vi "TestExplicitMessgaes.vi"() -> ()   [LabVIEW 2022 SP3, in "TopLevel.lvclass"]
uses:
  TopLevel/TopLevel.lvclass
  Typedefs/SetExplicitMessage API Data.ctl
  Typedefs/Motor Controller Parameter-Set.ctl
  <vilib>/ethernetip/ethernetip.llb/ethernetip.ctl
  C:/projects/Digilens_IPLC/Classes/Motor Controller/EEIP.dll
  EEIP.dll
  Motor Controller.lvclass
  <vilib>/ethernetip/ethernetip.lvlib
panel:
  in  "SendCmd 2":bool
  in  "SetExplicitMessage API Data LV":T1={"Motor Controller Parameter"=enum."Home Stage", "value"=0}
  out "Return":cluster{"size":i32, "GetAttributeSingle":u8[]}
  in  "SendCmd":bool
  in  "SetExplicitMessage API Data":T1={"Motor Controller Parameter"=enum."Home Stage", "value"=0}
  in  "OK":bool
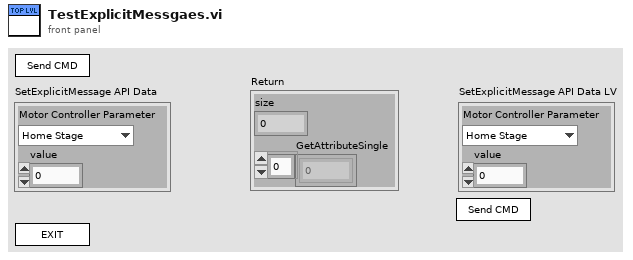
[diagram p1: front panel]
types:
  T1 = typedef "Motor Controller.lvclass/SetExplicitMessage API Data.ctl" = cluster{"Motor Controller Parameter":T2, "value":i32}
  T2 = typedef "Motor Controller.lvclass/Motor Controller Parameter-Set.ctl" = enum16{"Print Speed", "Jog Speed", "PR Path", "Enable Servo", "Disable Servo", "Move Stage to Under PH1", "Move Stage to Under PH2", "Move Stage to Under PH3", "Move Stage to Under PH4", "Move Stage to Under PH5", "Move Stage to Under PH6", "Home Stage", "Return Stage to 0", "Print Stage", "Write Speed", "Write Index", "Stop Stage"}
  T3 = enum32{"Invalid", "Standard", "Closed", "Hidden", "Minimized", "Maximized"}
  T4 = enum32{"invalid app kind", "Development System", "Run Time System", "Student Edition", "Embedded LabVIEW", "Evaluation", "Custom"}
  T5 = typedef "ethernetip.lvlib/ethernetip.ctl" = refnum<k21>
  T6 = cluster{"Core":cluster{"Current VI Reference":refnum<vi>, "Close Panel on Exit?":bool}, ".NET Refnum":refnum<k24>, "Session out":T5}
  T7 = cluster{"Current VI Reference":refnum<vi>, "Close Panel on Exit?":bool}
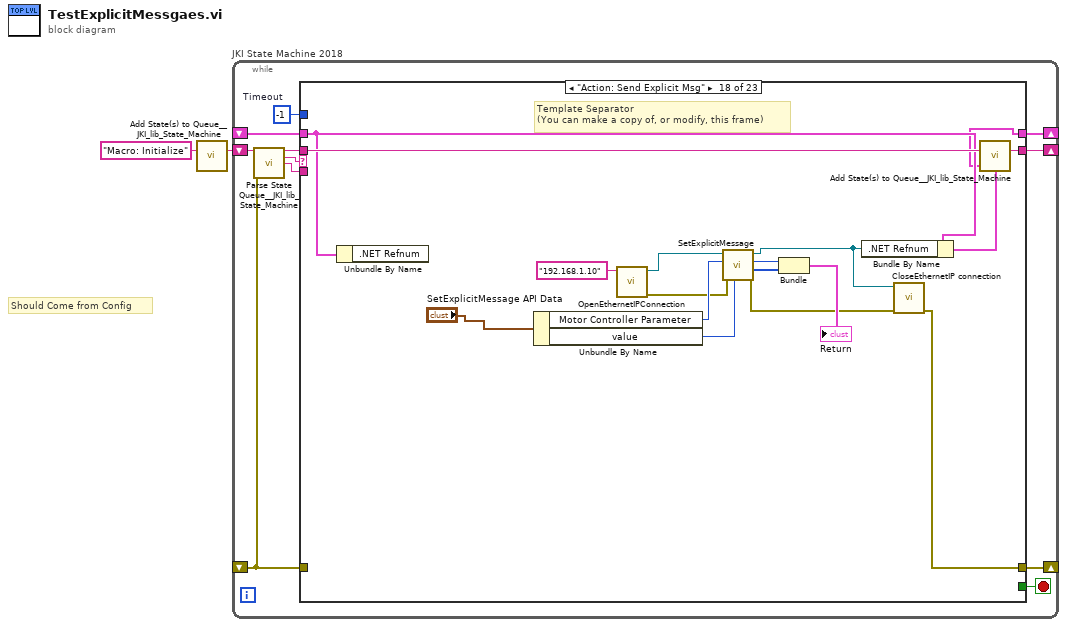
[diagram p0: block diagram]
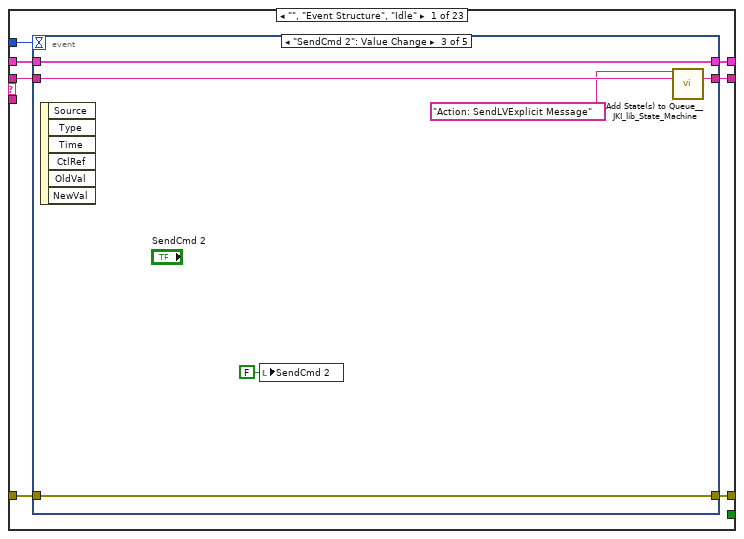
[diagram p2: hidden frame]
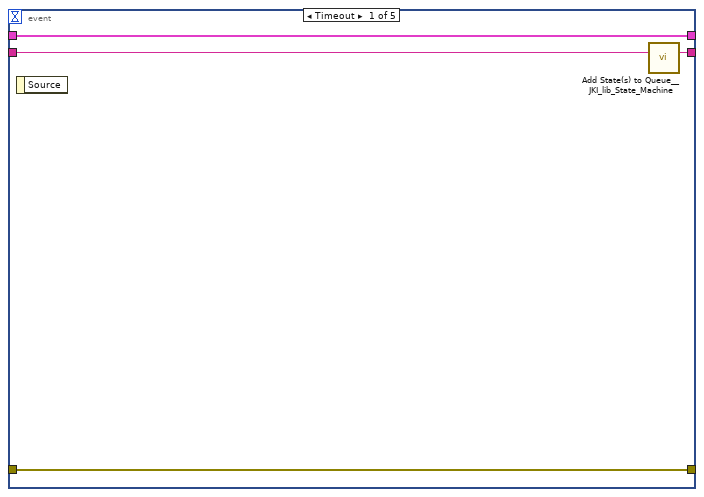
[diagram p3: hidden frame]
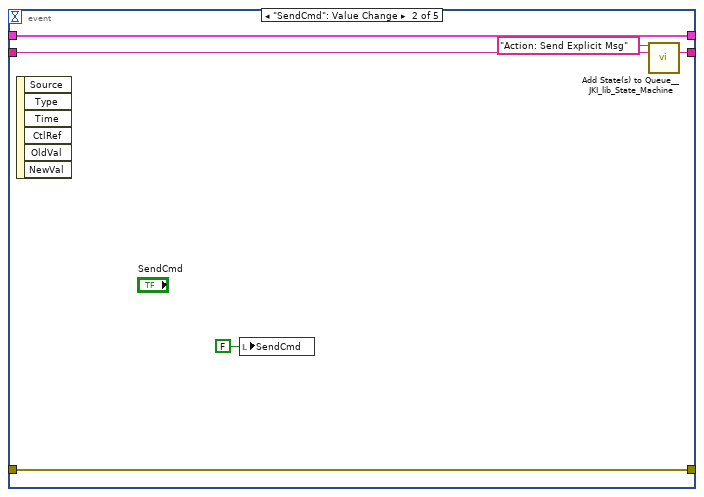
[diagram p4: hidden frame]
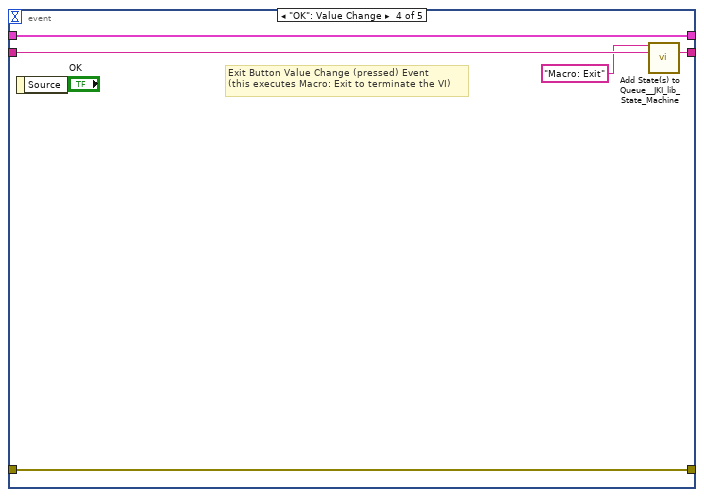
[diagram p5: hidden frame]
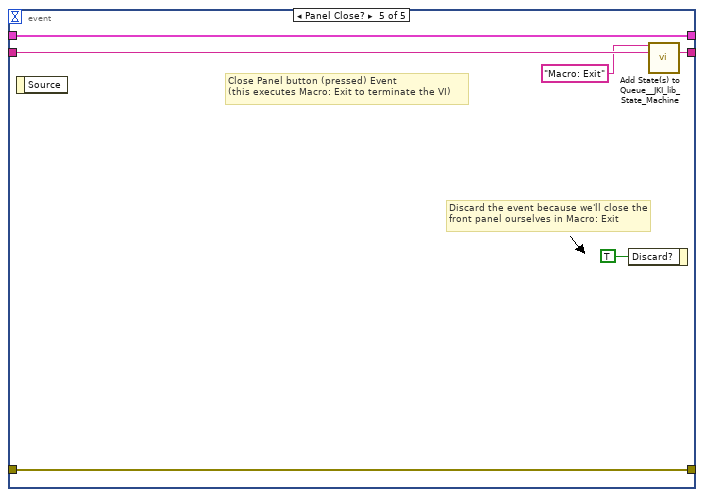
[diagram p6: hidden frame]
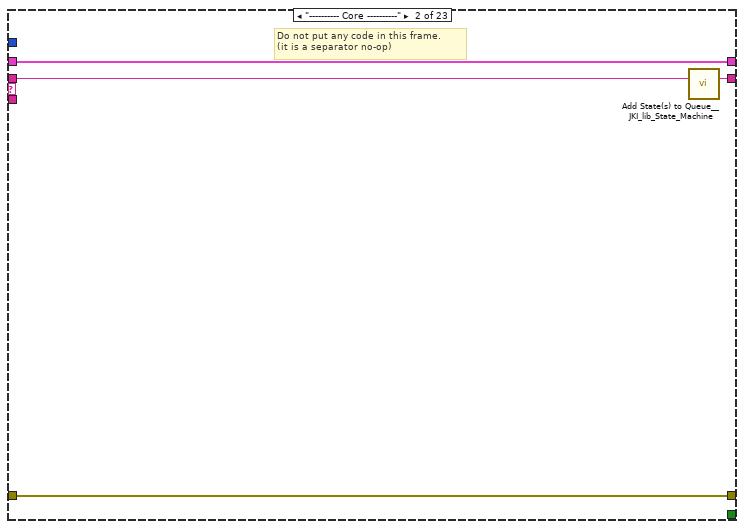
[diagram p7: hidden frame]
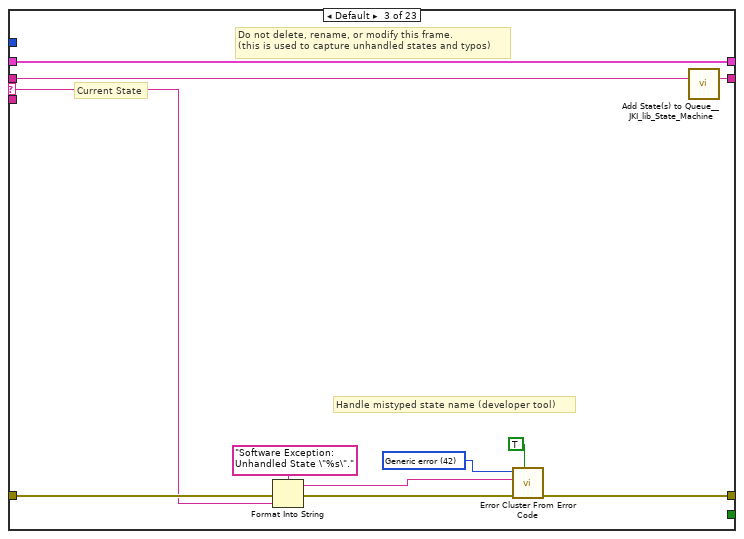
[diagram p8: hidden frame]
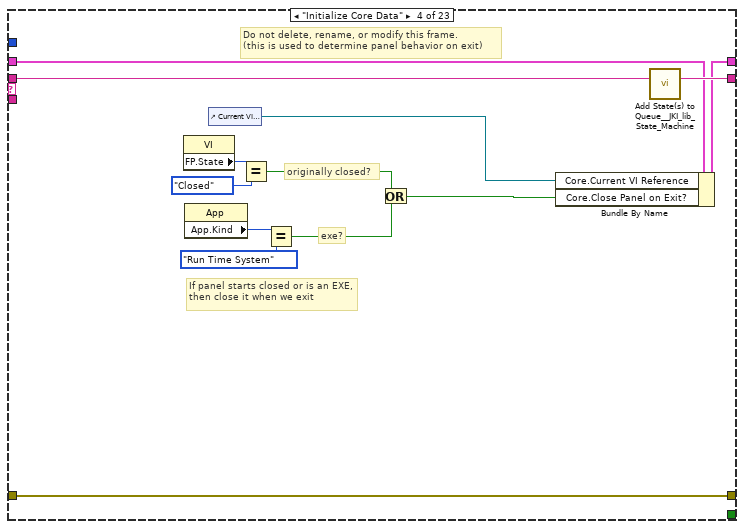
[diagram p9: hidden frame]
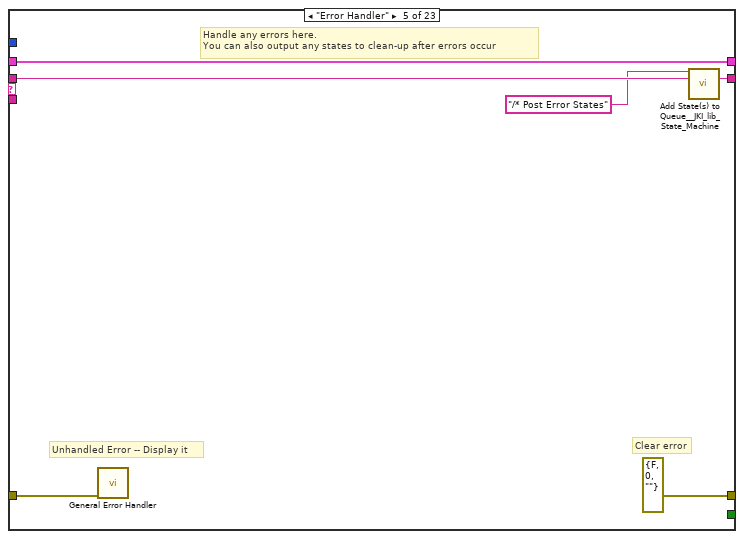
[diagram p10: hidden frame]
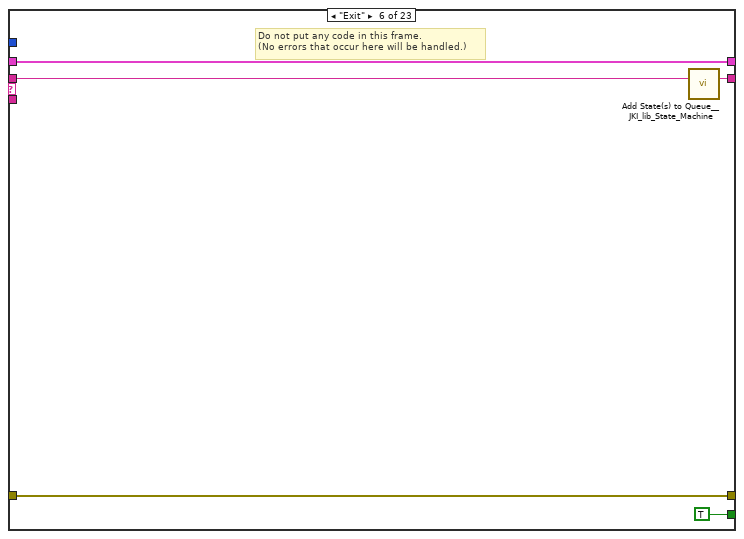
[diagram p11: hidden frame]
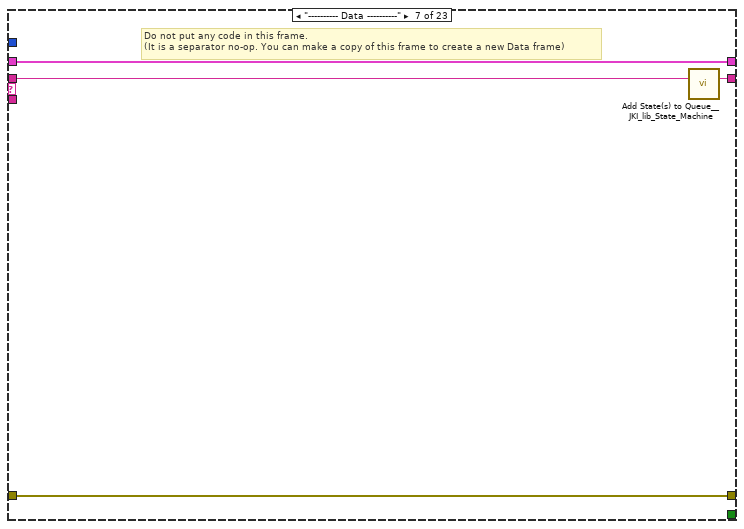
[diagram p12: hidden frame]
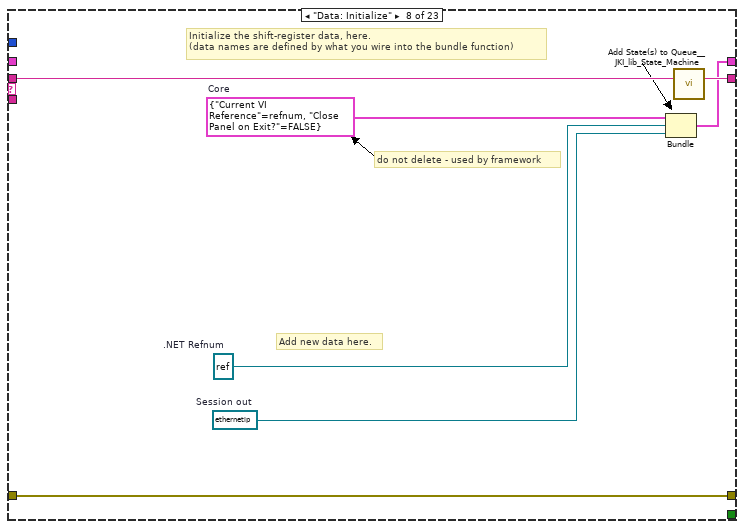
[diagram p13: hidden frame]
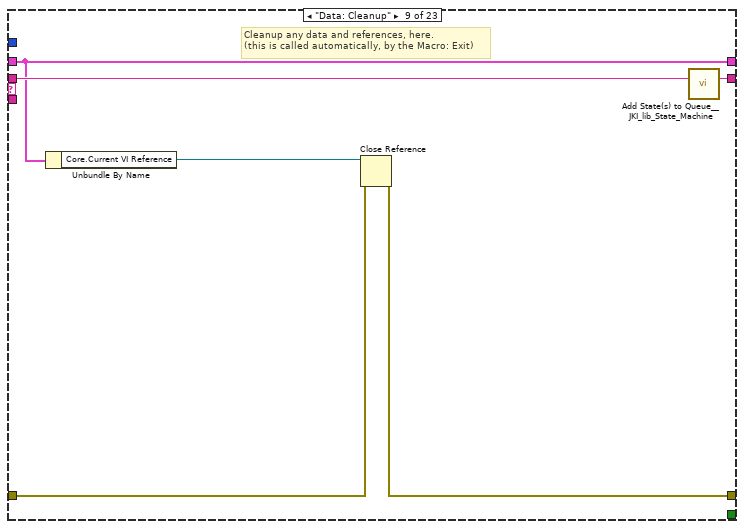
[diagram p14: hidden frame]
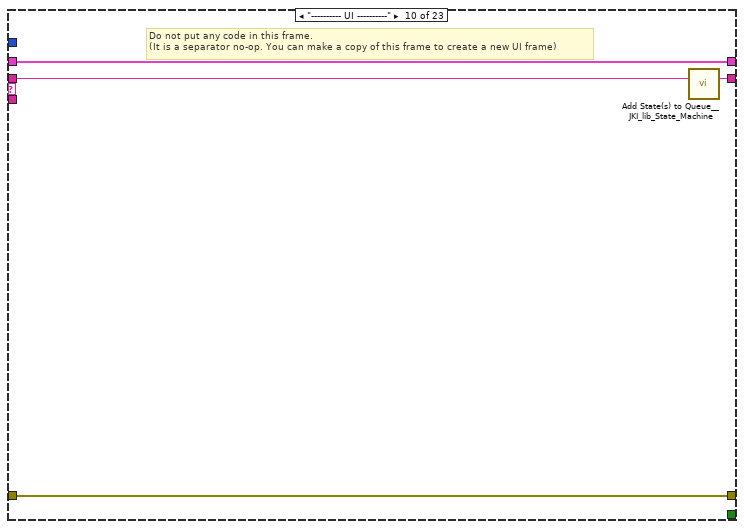
[diagram p15: hidden frame]
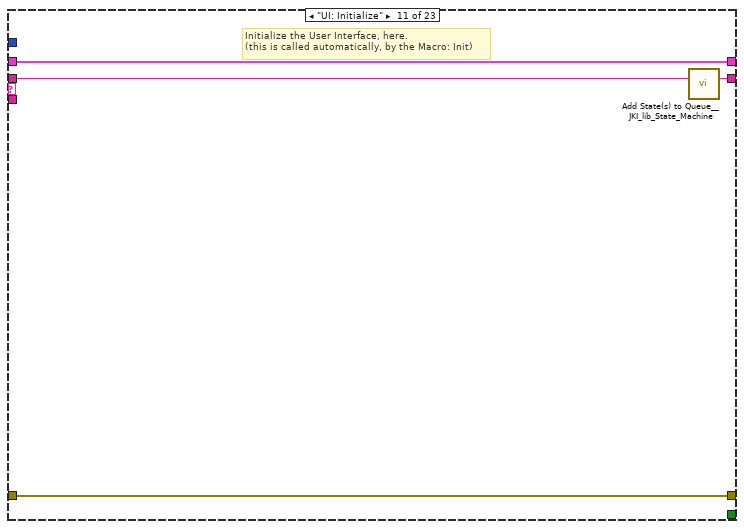
[diagram p16: hidden frame]
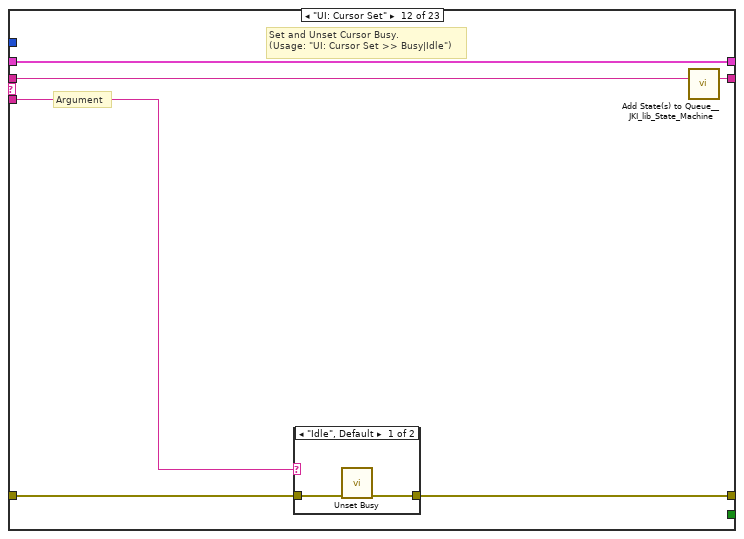
[diagram p17: hidden frame]
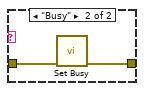
[diagram p18: hidden frame]
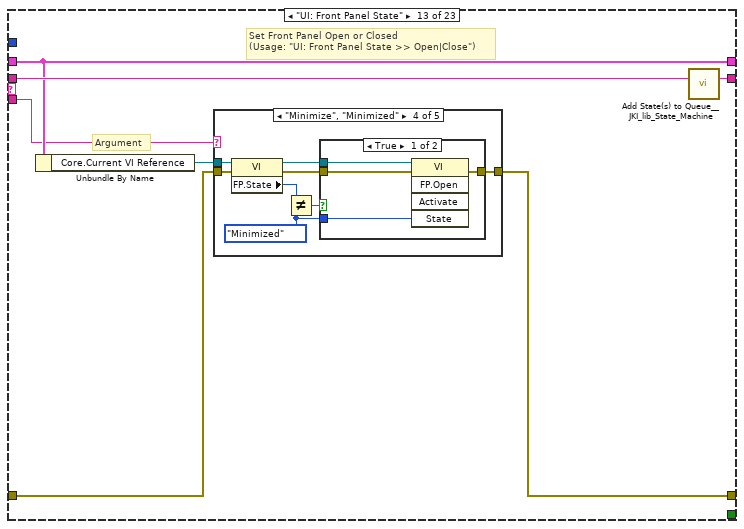
[diagram p19: hidden frame]
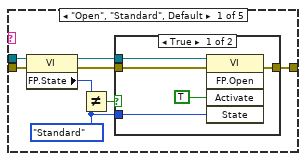
[diagram p20: hidden frame]
diagram:
  # "Should Come from Config"
  n1 = call <vilib>:"Add State(s) to Queue__JKI_lib_State_Machine.vi"("State(s) in (\"\")"="Macro: Initialize") -> ("States Out"=w2:string)  [unwired: 14 in]
  n2 = while "JKI State Machine 2018" {
    shift-right: [w6] -> _
    shift-left: _ -> [w5]
    shift-right: [w9] -> _
    shift-left: _ -> [w3]
    shift-right: [w8] -> _
    shift-left: w2 -> [w10]
    stop <- w7 stop-if-true
    w4 = -1  # Timeout
    n3 = call <vilib>:"Parse State Queue__JKI_lib_State_Machine.vi"("State Queue"=w10, "Error In (no error)"=w3) -> ("Remaining States"=w12:string, "Current State"=w13:string, "Arguments"=w11:string)  [unwired: 11 in]
    n4 = case shown="\"Action: Send Explicit Msg\"" w13 {
      selector: w13 -> [_ _ w52 _ _ _ _ _ _ _ _ _ _ _ _ _ _ _ _ _ _ _ _]
      tunnel: w12 -> [w20 w51 w56 w75 w81 w86 w90 w97 w103 w107 w111 w117 w128 w197 w202 w212 w216 w232 w243 w252 w261 w267 w273]
      tunnel: w11 -> [_ _ _ _ _ _ _ _ _ _ _ w112 w122 _ _ _ _ _ _ _ _ _ _]
      tunnel: w5 -> [w18 w48 w54 w68 w78 w84 w87 _ w98 w104 w109 w115 w124 w194 w199 w209 w213 w226 w241 w246 w258 w264 w271]
      tunnel: [w17 w49 w58 w72 errorcluster {"status"=FALSE, "code"=0, "source"=""} ("error out") w83 w88 w94 w99 w105 w108 w113 w125 w195 w200 w210 w214 w218 w236 w245 w257 w263 w268] -> w9
      tunnel: w3 -> [w16 w49 w57 w72 w77 w83 w88 w94 w100 w105 w108 w114 w126 w195 w200 w210 w214 _ w234 w244 w256 w262 w269]
      tunnel: [w19 w50 w55 w74 w80 w85 w89 w96 w102 w106 w110 w116 w127 w196 w201 w211 w215 w231 w242 w251 w260 w266 w272] -> w8
      tunnel: [_ _ _ _ _ TRUE _ _ _ _ _ _ _ _ _ _ _ _ _ _ _ _ _] -> w7
      tunnel: [w15 w48 w54 w73 w78 w84 w87 w95 w98 w104 w109 w115 w124 w194 w199 w209 w213 w225 w240 w247 w259 w264 w271] -> w6
      tunnel: w4 -> [w14 _ _ _ _ _ _ _ _ _ _ _ _ _ _ _ _ _ _ _ _ _ _]
      frame "", "Event Structure", "Idle" {
        n5 = event shown="[2] \"SendCmd 2\": Value Change" {
          selector: _ -> [_ _ _ _ _]
          dyn-events: _ -> [_ _ _ _ _]
          timeout: w14 -> [_ _ _ _ _]
          tunnel: w20 -> [w24 w30 w36 w41 w47]
          tunnel: [w23 w29 w35 w40 w46] -> w19
          tunnel: w18 -> [w21 w27 w33 w38 w44]
          tunnel: [w22 w28 w34 w39 w45] -> w17
          tunnel: w16 -> [w22 w28 w34 w39 w45]
          tunnel: [w21 w27 w33 w38 w44] -> w15
          event Timeout {
            n6 = event-data() -> ()  [unwired: 1 in, 1 out]
            n7 = call <vilib>:"Add State(s) to Queue__JKI_lib_State_Machine.vi"("State(s) in (\"\")"=w24) -> ("States Out"=w23:string)  [unwired: 14 in]
          }
          event "SendCmd": Value Change {
            n8 = event-data() -> ()  [unwired: 1 in, 6 out]
            n9 = local write "SendCmd"(FALSE ("SendCmd")) -> ()
            n10 = call <vilib>:"Add State(s) to Queue__JKI_lib_State_Machine.vi"("State(s) in Front (\"\")"="Action: Send Explicit Msg" ("State(s) in Front (\"\")"), "State(s) in (\"\")"=w30) -> ("States Out"=w29:string)  [unwired: 13 in]
          }
          event "SendCmd 2": Value Change {
            n11 = event-data() -> ()  [unwired: 1 in, 6 out]
            n12 = local write "SendCmd 2"(FALSE ("SendCmd")) -> ()
            n13 = call <vilib>:"Add State(s) to Queue__JKI_lib_State_Machine.vi"("State(s) in Front (\"\")"="Action: SendLVExplicit Message" ("State(s) in Front (\"\")"), "State(s) in (\"\")"=w36) -> ("States Out"=w35:string)  [unwired: 13 in]
          }
          event "OK": Value Change {
            # "Exit Button Value Change (pressed) Event\n(this executes Macro: Exit to terminate the VI)"
            n14 = event-data() -> ()  [unwired: 1 in, 1 out]
            n15 = call <vilib>:"Add State(s) to Queue__JKI_lib_State_Machine.vi"("State(s) in Front (\"\")"="Macro: Exit", "State(s) in (\"\")"=w41) -> ("States Out"=w40:string)  [unwired: 13 in]
          }
          event Panel Close? {
            # "Discard the event because we'll close the front panel ourselves in Macro: Exit"
            # "Close Panel button (pressed) Event\n(this executes Macro: Exit to terminate the VI)"
            n16 = event-data() -> ()  [unwired: 1 in, 1 out]
            n17 = event-data("Discard?"=TRUE) -> ()  [unwired: 1 in, 1 out]
            n18 = call <vilib>:"Add State(s) to Queue__JKI_lib_State_Machine.vi"("State(s) in Front (\"\")"="Macro: Exit", "State(s) in (\"\")"=w47) -> ("States Out"=w46:string)  [unwired: 13 in]
          }
        }
      }
      frame "---------- Core ----------" {
        # "Do not put any code in this frame.\n(it is a separator no-op)"
        n19 = call <vilib>:"Add State(s) to Queue__JKI_lib_State_Machine.vi"("State(s) in (\"\")"=w51) -> ("States Out"=w50:string)  [unwired: 14 in]
      }
      frame Default {
        w61 = 42 items=["No error", "Argument error", "Memory is full", "Out of zone", "End of file", "File already open", "Generic file I/O error", "File not found", "File permission error", "Disk is full", "Duplicate path", "Too many files open", "System feature not enabled", "Resource file not found", "Cannot add resource", "Resource not found", "Image not found", "Image memory error", "Pen does not exist", "Config type invalid", "Config token not found", "Config parse error", "Config memory error", "Bad external code format", "Bad external code offset", "External code not present", "Null window", "Destroy window error", "Null menu", "Print aborted", "Bad print record", "Print driver error", "Windows error during printing", "Memory error during printing", "Print dialog error", "Generic print error", "Invalid device refnum", "Device not found", "Device parameter error", "Device unit error", "Cannot open device", "Device call aborted", "Generic error", "Cancelled by user", "Object ID too low", "Object ID too high", "Object not in heap", "Unknown heap", "Unknown object (invalid DefProc)", "Unknown object (DefProc not in table)", "Message out of range", "Invalid (null) method", "Unknown message", "Manager call not supported", "Bad address", "Network operation in progress", "Network operation timed out", "Connection is busy", "Network attribute not supported", "Network error", "Address in use", "System out of memory", "Connection aborted", "Connection refused", "Not connected", "Already connected", "Connection closed", "Initialization error (interapplication manager)", "Bad occurrence", "Wait on unbound occurrence handler", "Occurrence queue overflow", "Datalog type conflict", "Unused", "Unrecognized type (interapplication manager)", "Memory corrupt", "Failed to make temporary DLL", "Old CIN version", "Drag socket not found", "Failed to load drop-object", "Failed to register OLE object", "Failed to release OLE object", "Format specifier type mismatch", "Unknown format specifier", "Too few format specifiers", "Too many format specifiers", "Scan failed", "Newer CIN version", "Error converting to variant", "Runtime menu error", "Password tampered", "Variant attribute not found", "Incompatible variant data type", "Event data is not available", "Event Store is not present", "Occurrence is not found", "Event Queue is not created", "Event info is not available", "Refnum passed is NULL", "Error retrieving Class GUID", "Error retrieving CoClass GUID", "Error retrieving TypeLib GUID.", "Bad built application magic bytes.", "Specific driver is different from the specific driver associated with the Logical Name.", "There is no session opened to the class driver.", "Max Error", "MAX - Error with config objects", "MAX - Error loading configuration", "MAX - Group not supported"]
        # "Current State"
        # "Do not delete, rename, or modify this frame.\n(this is used to capture unhandled states and typos)"
        # "Handle mistyped state name (developer tool)"
        n20 = Format Into String(format string="Software Exception: Unhandled State \"%s\"." ("message"), error in=w57, w52) -> (resulting string=w60:string, error out=w59:errorcluster)  [unwired: 1 in]
        n21 = call <vilib>:"Error Cluster From Error Code.vi"("show call chain? (False)"=TRUE, "error in (no error)"=w59, "error message (\"\")"=w60, "error code (0)"=w61) -> ("error out"=w58:errorcluster)  [unwired: 5 in]
        n22 = call <vilib>:"Add State(s) to Queue__JKI_lib_State_Machine.vi"("State(s) in (\"\")"=w56) -> ("States Out"=w55:string)  [unwired: 14 in]
      }
      frame "Initialize Core Data" {
        # "Do not delete, rename, or modify this frame.\n(this is used to determine panel behavior on exit)"
        # "originally closed?"
        # "exe?"
        # "If panel starts closed or is an EXE, then close it when we exit"
        n23 = property class="VI"() -> ("FP.State"=w65:T3)  [unwired: 2 in, 2 out]
        n24 = property class="App"() -> ("App.Kind"=w71:T4)  [unwired: 2 in, 2 out]
        n25 = control-ref of="Current VI Reference"() -> (w66:refnum<vi>)
        n26 = Equal?(x=w65, y=T3."Closed" ("Front Panel Window:State")) -> (x = y?=w63:bool)
        n27 = Equal?(x=w71, y=T4."Run Time System" ("Application:Kind")) -> (x = y?=w69:bool)
        n28 = Or(x=w63, y=w69) -> (x .or. y?=w67:bool)
        n29 = Bundle By Name(cluster=w68, "Core.Current VI Reference"=w66, "Core.Close Panel on Exit?"=w67) -> (w73:T6)
        n30 = call <vilib>:"Add State(s) to Queue__JKI_lib_State_Machine.vi"("State(s) in (\"\")"=w75) -> ("States Out"=w74:string)  [unwired: 14 in]
      }
      frame "Error Handler" {
        # "Unhandled Error -- Display it"
        # "Handle any errors here.\nYou can also output any states to clean-up after errors occur"
        # "Clear error"
        n31 = call <vilib>:"General Error Handler.vi"("error in (no error)"=w77) -> ()  [unwired: 10 in, 5 out]
        n32 = call <vilib>:"Add State(s) to Queue__JKI_lib_State_Machine.vi"("State(s) in Front (\"\")"="/* Post Error States", "State(s) in (\"\")"=w81) -> ("States Out"=w80:string)  [unwired: 13 in]
      }
      frame "Exit" {
        # "Do not put any code in this frame.\n(No errors that occur here will be handled.)"
        n33 = call <vilib>:"Add State(s) to Queue__JKI_lib_State_Machine.vi"("State(s) in (\"\")"=w86) -> ("States Out"=w85:string)  [unwired: 14 in]
      }
      frame "---------- Data ----------" {
        # "Do not put any code in this frame.\n(It is a separator no-op. You can make a copy of this frame to create a new Data frame)"
        n34 = call <vilib>:"Add State(s) to Queue__JKI_lib_State_Machine.vi"("State(s) in (\"\")"=w90) -> ("States Out"=w89:string)  [unwired: 14 in]
      }
      frame "Data: Initialize" {
        w91 = T5 refnum  # Session out
        w92 = refnum<k24> refnum  # .NET Refnum
        w93 = T7 {"Current VI Reference"=refnum, "Close Panel on Exit?"=FALSE}  # Core
        # "do not delete - used by framework"
        # "Add new data here."
        # "Initialize the shift-register data, here.\n(data names are defined by what you wire into the bundle function)"
        n35 = Bundle("Core"=w93, ".NET Refnum"=w92, "Session out"=w91) -> (w95:T6)  [unwired: 1 in]
        n36 = call <vilib>:"Add State(s) to Queue__JKI_lib_State_Machine.vi"("State(s) in (\"\")"=w97) -> ("States Out"=w96:string)  [unwired: 14 in]
      }
      frame "Data: Cleanup" {
        # "Cleanup any data and references, here.\n(this is called automatically, by the Macro: Exit)"
        n37 = Unbundle By Name(w98) -> ("Core.Current VI Reference"=w101:refnum<vi>)
        n38 = Close Reference(reference=w101, error in (no error)=w100) -> (error out=w99:errorcluster)
        n39 = call <vilib>:"Add State(s) to Queue__JKI_lib_State_Machine.vi"("State(s) in (\"\")"=w103) -> ("States Out"=w102:string)  [unwired: 14 in]
      }
      frame "---------- UI ----------" {
        # "Do not put any code in this frame.\n(It is a separator no-op. You can make a copy of this frame to create a new UI frame)"
        n40 = call <vilib>:"Add State(s) to Queue__JKI_lib_State_Machine.vi"("State(s) in (\"\")"=w107) -> ("States Out"=w106:string)  [unwired: 14 in]
      }
      frame "UI: Initialize" {
        # "Initialize the User Interface, here.\n(this is called automatically, by the Macro: Init)"
        n41 = call <vilib>:"Add State(s) to Queue__JKI_lib_State_Machine.vi"("State(s) in (\"\")"=w111) -> ("States Out"=w110:string)  [unwired: 14 in]
      }
      frame "UI: Cursor Set" {
        # "Argument"
        # "Set and Unset Cursor Busy.\n(Usage: \"UI: Cursor Set >> Busy|Idle\")"
        n42 = case shown="\"Idle\", Default" w112 {
          tunnel: w114 -> [w119 w121]
          tunnel: [w118 w120] -> w113
          frame "Idle", Default {
            n43 = call <vilib>:"Unset Busy.vi"("error in (no error)"=w119) -> ("error out"=w118:errorcluster)  [unwired: 10 in]
          }
          frame "Busy" {
            n44 = call <vilib>:"Set Busy.vi"("error in (no error)"=w121) -> ("error out"=w120:errorcluster)  [unwired: 9 in, 1 out]
          }
        }
        n45 = call <vilib>:"Add State(s) to Queue__JKI_lib_State_Machine.vi"("State(s) in (\"\")"=w117) -> ("States Out"=w116:string)  [unwired: 14 in]
      }
      frame "UI: Front Panel State" {
        # "Argument"
        # "Set Front Panel Open or Closed\n(Usage: \"UI: Front Panel State >> Open|Close\")"
        n46 = Unbundle By Name(w124) -> ("Core.Current VI Reference"=w123:refnum<vi>)
        n47 = case shown="\"Minimize\", \"Minimized\"" w122 {
          tunnel: w126 -> [w134 w149 w160 w173 w186]
          tunnel: [w136 w150 w162 w175 w188] -> w125
          tunnel: w123 -> [w135 w147 w161 w174 w187]
          frame "Open", "Standard", Default {
            w129 = T3."Standard" ("State")
            n48 = property class="VI"(reference=w135, error in=w134) -> (reference out=w132:refnum<vi>, error out=w133:errorcluster, "FP.State"=w131:T3)
            n49 = Not Equal?(x=w131, y=w129) -> (x != y?=w130:bool)
            n50 = case shown="True" w130 {
              tunnel: [w140 w142] -> w136
              tunnel: w133 -> [w139 w142]
              tunnel: w132 -> [w138 _]
              tunnel: w129 -> [w137 _]
              frame True {
                n51 = invoke class="VI" method="FP.Open"(reference=w138, error in=w139, "Activate"=TRUE, "State"=w137) -> (error out=w140:errorcluster)  [unwired: 1 in, 4 out]
              }
              frame False {
              }
            }
          }
          frame "Close", "Closed" {
            n52 = property class="VI"(reference=w147, error in=w149) -> (reference out=w146:refnum<vi>, error out=w148:errorcluster, "FP.State"=w144:T3)
            n53 = Not Equal?(x=w144, y=T3."Closed" ("Front Panel Window:State")) -> (x != y?=w143:bool)
            n54 = case shown="True" w143 {
              tunnel: [w151 w154] -> w150
              tunnel: w148 -> [w151 w153]
              tunnel: w146 -> [_ w152]
              frame False {
              }
              frame True {
                n55 = invoke class="VI" method="FP.Close"(reference=w152, error in=w153) -> (error out=w154:errorcluster)  [unwired: 1 in, 2 out]
              }
            }
          }
          frame "Hidden", "Hide" {
            w155 = T3."Hidden" ("State")
            n56 = property class="VI"(reference=w161, error in=w160) -> (reference out=w158:refnum<vi>, error out=w159:errorcluster, "FP.State"=w157:T3)
            n57 = Not Equal?(x=w157, y=w155) -> (x != y?=w156:bool)
            n58 = case shown="True" w156 {
              tunnel: [w166 w167] -> w162
              tunnel: w159 -> [w165 w167]
              tunnel: w158 -> [w164 _]
              tunnel: w155 -> [w163 _]
              frame True {
                n59 = invoke class="VI" method="FP.Open"(reference=w164, error in=w165, "State"=w163) -> (error out=w166:errorcluster)  [unwired: 2 in, 4 out]
              }
              frame False {
              }
            }
          }
          frame "Minimize", "Minimized" {
            w168 = T3."Minimized" ("State")
            n60 = property class="VI"(reference=w174, error in=w173) -> (reference out=w171:refnum<vi>, error out=w172:errorcluster, "FP.State"=w170:T3)
            n61 = Not Equal?(x=w170, y=w168) -> (x != y?=w169:bool)
            n62 = case shown="True" w169 {
              tunnel: [w179 w180] -> w175
              tunnel: w172 -> [w178 w180]
              tunnel: w171 -> [w177 _]
              tunnel: w168 -> [w176 _]
              frame True {
                n63 = invoke class="VI" method="FP.Open"(reference=w177, error in=w178, "State"=w176) -> (error out=w179:errorcluster)  [unwired: 2 in, 4 out]
              }
              frame False {
              }
            }
          }
          frame "Maximize", "Maximized" {
            w181 = T3."Maximized" ("State")
            n64 = property class="VI"(reference=w187, error in=w186) -> (reference out=w184:refnum<vi>, error out=w185:errorcluster, "FP.State"=w183:T3)
            n65 = Not Equal?(x=w183, y=w181) -> (x != y?=w182:bool)
            n66 = case shown="True" w182 {
              tunnel: [w192 w193] -> w188
              tunnel: w185 -> [w191 w193]
              tunnel: w184 -> [w190 _]
              tunnel: w181 -> [w189 _]
              frame True {
                n67 = invoke class="VI" method="FP.Open"(reference=w190, error in=w191, "State"=w189) -> (error out=w192:errorcluster)  [unwired: 2 in, 4 out]
              }
              frame False {
              }
            }
          }
        }
        n68 = call <vilib>:"Add State(s) to Queue__JKI_lib_State_Machine.vi"("State(s) in (\"\")"=w128) -> ("States Out"=w127:string)  [unwired: 14 in]
      }
      frame "---------- Macro ----------" {
        # "Do not put any code in this frame.\n(It is a separator no-op. You can make a copy of this frame to create a new Macro frame)"
        n69 = call <vilib>:"Add State(s) to Queue__JKI_lib_State_Machine.vi"("State(s) in (\"\")"=w197) -> ("States Out"=w196:string)  [unwired: 14 in]
      }
      frame "Macro: Initialize" {
        w198 = "Data: Initialize\nInitialize Core Data\nUI: Initialize\n/*Connection: Open\nConnection2: Open\nUI: Front Panel State >> Open"  # Data: Initialize Initialize Core Data UI: Initialize /*Connection: Open Connection2: Open UI: Front Panel State >> Open
        # "Initialization Macro\n(This is called once, when the VI starts)"
        n70 = call <vilib>:"Add State(s) to Queue__JKI_lib_State_Machine.vi"("State(s) in Front (\"\")"=w198, "State(s) in (\"\")"=w202) -> ("States Out"=w201:string)  [unwired: 13 in]
      }
      frame "Macro: Exit" {
        # "Exit Macro\n(This is called once, when the VI exits)"
        n71 = Unbundle By Name(w209) -> ("Core.Close Panel on Exit?"=w208:bool)
        n72 = Select(t="UI: Front Panel State >> Close", s=w208, f="") -> (s? t:f=w205:string)
        n73 = call <vilib>:"Add State(s) to Queue__JKI_lib_State_Machine.vi"("State(s) in (\"\")"=w205, "State(s) at Back (\"\")"="/*Connection: Close\nConnection2: Close\nData: Cleanup\nExit") -> ("States Out"=w203:string)  [unwired: 13 in]
        n74 = call <vilib>:"Add State(s) to Queue__JKI_lib_State_Machine.vi"("State(s) in Front (\"\")"=w203, "State(s) in (\"\")"=w212) -> ("States Out"=w211:string)  [unwired: 13 in]
      }
      frame "---------- New Category ----------" {
        # "Template Separator\n(You can make a copy of, or modify, this frame)"
        n75 = call <vilib>:"Add State(s) to Queue__JKI_lib_State_Machine.vi"("State(s) in (\"\")"=w216) -> ("States Out"=w215:string)  [unwired: 14 in]
      }
      frame "Action: Send Explicit Msg" {
        # "Template Separator\n(You can make a copy of, or modify, this frame)"
        n76 = Unbundle By Name(w226) -> ()  [unwired: 1 out]
        n77 = Unbundle By Name("SetExplicitMessage API Data") -> ("Motor Controller Parameter"=w228:T2, "value"=w227:i32)
        n78 = call "OpenEthernetIPConnection.vi"("String"="192.168.1.10") -> ("error out"=w217:errorcluster, ".NET Refnum out"=w221:refnum<k24>)  [unwired: 9 in]
        n79 = call "SetExplicitMessage.vi"("value"=w227, "error in (no error)"=w217, "Motor Controller Parameter"=w228, ".NET Refnum in"=w221) -> ("error out"=w219:errorcluster, "GetAttributeSingle"=w229:u8[], "size"=w230:i32, ".NET Refnum out"=w220:refnum<k24>)  [unwired: 3 in, 1 out]
        n80 = Bundle("size"=w230, "GetAttributeSingle"=w229) -> (→"Return":cluster{"size":i32, "GetAttributeSingle":u8[]})  [unwired: 1 in]
        n81 = Bundle By Name(cluster=w226, ".NET Refnum"=w220) -> (w225:T6)
        n82 = call "CloseEthernetIP connection.vi"("error in (no error)"=w219, ".NET Refnum in"=w220) -> ("error out"=w218:errorcluster)  [unwired: 9 in]
        n83 = call <vilib>:"Add State(s) to Queue__JKI_lib_State_Machine.vi"("State(s) in (\"\")"=w232) -> ("States Out"=w231:string)  [unwired: 14 in]
      }
      frame "Action: SendLVExplicit Message" {
        # "Template Separator\n(You can make a copy of, or modify, this frame)"
        n84 = Unbundle By Name("SetExplicitMessage API Data LV") -> ("Motor Controller Parameter"=w238:T2, "value"=w235:i32)
        n85 = Unbundle By Name(w241) -> ("Session out"=w233:T5)
        n86 = call "SendLVEthIP_ExplicitMessage.vi"("error in (no error)"=w234, "value"=w235, "Motor Controller Parameter"=w238, "Refnum in"=w233) -> ("error out"=w236:errorcluster, "Refnum out"=w237:T5)  [unwired: 6 in]
        n87 = Bundle By Name(cluster=w241, "Session out"=w237) -> (w240:T6)
        n88 = call <vilib>:"Add State(s) to Queue__JKI_lib_State_Machine.vi"("State(s) in (\"\")"=w243) -> ("States Out"=w242:string)  [unwired: 14 in]
      }
      frame "Connection: Open" {
        # "Should Come from Config"
        # "Your code here.\n(You can make a copy of, or modify, this frame)"
        n89 = call "OpenEthernetIPConnection.vi"("String"="192.168.1.10") -> ("error out"=w249:errorcluster, ".NET Refnum out"=w248:refnum<k24>)  [unwired: 9 in]
        n90 = Bundle By Name(cluster=w246, ".NET Refnum"=w248) -> (w247:T6)
        n91 = Merge Errors(w244, w249) -> (w245:errorcluster)
        n92 = call <vilib>:"Add State(s) to Queue__JKI_lib_State_Machine.vi"("State(s) in (\"\")"=w252) -> ("States Out"=w251:string)  [unwired: 14 in]
      }
      frame "Connection2: Open" {
        # "Should Come from Config"
        # "Your code here.\n(You can make a copy of, or modify, this frame)"
        n93 = call <vilib>:"EthernetIP Open Session.vi"("Session in"="192.168.1.10" ("String")) -> ("error out"=w254:errorcluster, "Session out"=w253:T5)  [unwired: 9 in]
        n94 = Bundle By Name(cluster=w258, "Session out"=w253) -> (w259:T6)
        n95 = Merge Errors(w256, w254) -> (w257:errorcluster)
        n96 = call <vilib>:"Add State(s) to Queue__JKI_lib_State_Machine.vi"("State(s) in (\"\")"=w261) -> ("States Out"=w260:string)  [unwired: 14 in]
      }
      frame "Connection: Close" {
        # "Your code here.\n(You can make a copy of, or modify, this frame)"
        n97 = Unbundle By Name(w264) -> (".NET Refnum"=w265:refnum<k24>)
        n98 = call "CloseEthernetIP connection.vi"("error in (no error)"=w262, ".NET Refnum in"=w265) -> ("error out"=w263:errorcluster)  [unwired: 9 in]
        n99 = call <vilib>:"Add State(s) to Queue__JKI_lib_State_Machine.vi"("State(s) in (\"\")"=w267) -> ("States Out"=w266:string)  [unwired: 14 in]
      }
      frame "Connection2: Close" {
        # "Your code here.\n(You can make a copy of, or modify, this frame)"
        n100 = Unbundle By Name(w271) -> ("Session out"=w270:T5)
        n101 = call <vilib>:"EthernetIP Close Session.vi"("error in"=w269, "Session in"=w270) -> ("error out"=w268:errorcluster)  [unwired: 9 in]
        n102 = call <vilib>:"Add State(s) to Queue__JKI_lib_State_Machine.vi"("State(s) in (\"\")"=w273) -> ("States Out"=w272:string)  [unwired: 14 in]
      }
    }
  }
